vi "Generation and Filter (FPGA).vi"() -> ()   [LabVIEW 2016]
doc: "This VI supports an application to generate, output, measure, and filter a waveform. It generates a clean sine wave, adds white noise to simulate a noisy measurement and writes it to analog output AO0 on the sbRIO evaluation board.\n\nThe signal is then read in through analog input AI22. While data is read, it is passed through an FPGA butterworth filter to remove the added white noise and reconstruct the clean sine wave.\n\nHardware Connection Fulfilled - Analog Output 0 is internally connected to Analog Input 22 via internal board routing.\nModA and ModB properties have been configured for Raw (I16) measurements instead of the default Callibrated (fixed-point) measurements."
uses:
  <vilib>/rvi/Emulation/niFpgaGetClockAttributes.vi
  <vilib>/rvi/Emulation/niFpgaSctlEmulationGetInTimedLoop.vi
  <vilib>/rvi/Emulation/niFpgaEmulationReportErrorSimple.vi
  <vilib>/rvi/eio/common/nirviEmuTemplateMethod_errors.vi
  <vilib>/rvi/Emulation/niFpgaCriticalErrorInLSC.vi
  <vilib>/eio/EIONode/EIONode.xnode
  <vilib>/rvi/Analysis/measure/butterworth/XNode/niFpgaButterworthFilter.xnode
panel:
  out "Clean Sine":i16
  out "Measured Sine":i16
  out "Filtered Sine":i16
  out "Noisy Sine":i16
  # "This application generates, outputs, measures, and filters a waveform. \nIt generates a clean sine wave, adds white noise to simulate a noisy \nmeasurement, and writes it to analog output AO0 on the evaluation board.\n\nThe signal is then read in through analog input AI1.  While data is read, it is \npassed through a butterworth filter implimented on the FPGA to remove the \nadded white noise and reconstruct the clean sine wave.\n\nHardware Connection - Analog Output 0 (AO0) must be physically wired\nto Analog Input 0 (AI0) via daughtercard terminals. ModA and ModB \nproperties have been configured for Raw (I16) measurements instead of\nthe default Calibrated (fixed-point) measurements."
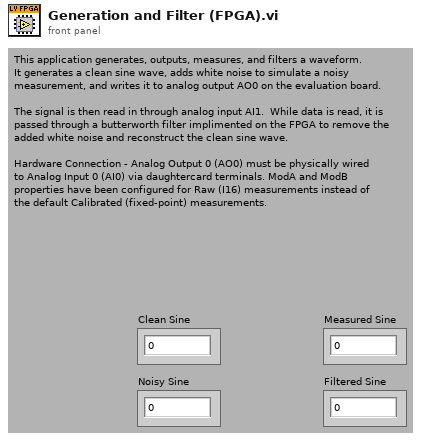
[diagram p1: front panel]
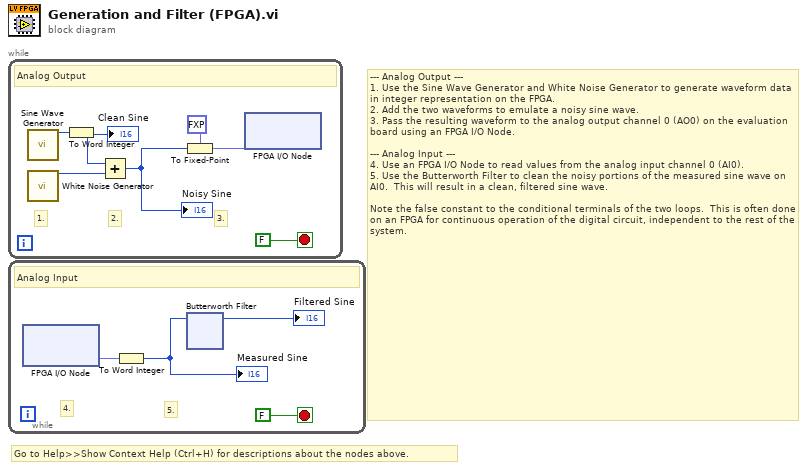
[diagram p0: block diagram]
diagram:
  # "Go to Help>>Show Context Help (Ctrl+H) for descriptions about the nodes above."
  # "--- Analog Output ---\n1. Use the Sine Wave Generator and White Noise Generator to generate waveform data in integer representation on the FPGA.\n2. Add the two waveforms to emulate a noisy sine wave.\n3. Pass the resulting waveform to the analog output channel 0 (AO0) on the evaluation board using an FPGA I/O Node.\n\n--- Analog Input ---\n4. Use an FPGA I/O Node to read values from the analog input channel 0 (AI0).  \n5. Use the Butterworth Filter to clean the noisy portions of the measured sine wave on AI0.  This will result in a clean, filtered sine wave.\n\nNote the false constant to the conditional terminals of the two loops.  This is often done on an FPGA for continuous operation of the digital circuit, independent to the rest of the system."
  n1 = while {
    stop <- FALSE stop-if-true
    # "3."
    # "2."
    # "1."
    # "Analog Output"
    n2 = call "Sine Wave Generator"() -> ("sine out"=w2:i8)  [unwired: 15 in]
    n3 = call "White Noise Generator"() -> ("white noise out"=w7:i16)  [unwired: 2 in, 13 out]
    n4 = To Word Integer(number=w2) -> (16bit integer=w1:i16)
    "Clean Sine" <- w1
    n5 = Add(x=w1, y=w7) -> (x+y=w5:i16)
    "Noisy Sine" <- w5
    n6 = To Fixed-Point(fixed-point type=fxp<+/-,20,5> 0.0 ("AO0"), number=w5) -> (fixed-point=w3:fxp<+/-,20,5>)
    n7 = xnode "FPGA I/O Node"("AO0"=w3) -> ()  [unwired: 1 in, 1 out]
  }
  n8 = while {
    stop <- FALSE stop-if-true
    # "5."
    # "4."
    # "Analog Input"
    n9 = xnode "FPGA I/O Node"() -> ("AI0"=w9:fxp<+/-,24,5>)  [unwired: 2 in, 2 out]
    n10 = To Word Integer(number=w9) -> (16bit integer=w8:i16)
    "Measured Sine" <- w8
    n11 = xnode "Butterworth Filter"("input data"=w8) -> ("output data"=→"Filtered Sine":i16)  [unwired: 2 in]
  }
